vi "Test MIO Digital Measurement.vi"(7 "Config":T1={"Samples to Read (50)"=50, "Channel (0)"=0, "Read Function (Get All)"=enum."Get Latest", "Port(0)"=0}, 8 "error in (no error)":errorcluster, 9 "Instrument":i32, 10 "Test Label":string, 11 "Test Class in":refnum<class "Test Class.lvclass">) -> (0 "error out":errorcluster, 1 "Result":string, 2 "Passed":bool, 3 "Test Class out":refnum<class "Test Class.lvclass">)   [LabVIEW 2015, in "Test Class.lvclass"]
uses:
  Test Class.lvclass
  Digital MIO Measurement Config -- Cluster.ctl
  Classes/Instruments/MIO Device/Class/typedefs/Read Type -- Enum.ctl
  Classes/Instruments/MIO Device/Class/typedefs/Channel Type -- Enum.ctl
  Classes/Instruments/MIO Device/Class/MIO Device.lvclass
  Test Class.lvclass/Test Class.ctl
  Classes/Application/Class/Application.lvclass
  Classes/Test Recipe/Class/Test Recipe.lvclass
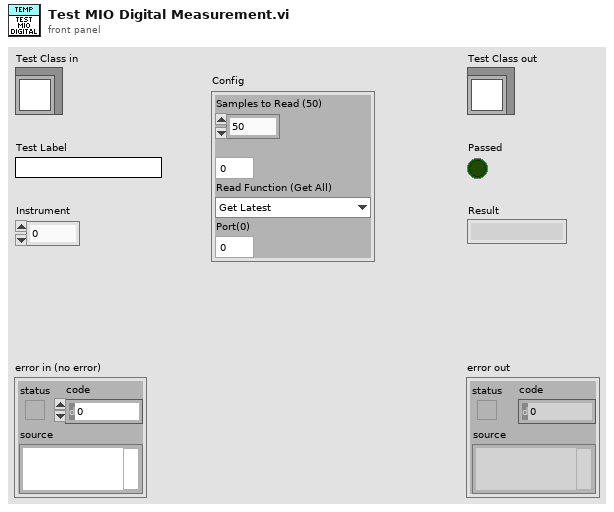
[diagram p1: front panel]
types:
  T1 = typedef "Test Class.lvclass/Digital MIO Measurement Config -- Cluster.ctl" = cluster{"Samples to Read (50)":i32, "Channel (0)":u32, "Read Function (Get All)":T2, "Port(0)":u32}
  T2 = typedef "MIO Device.lvlib/MIO Device.lvclass/Read Type -- Enum.ctl" = enum16{"Get All", "Get Latest", "Get Average"}
  T3 = typedef "MIO Device.lvlib/MIO Device.lvclass/Channel Type -- Enum.ctl" = enum16{"Analog Input", "Analog Output", "Digital Input", "Digital Output"}
  T4 = typedef "Application.lvlib/App Properties.lvclass/Class Properties -- Cluster.ctl" = cluster{"UUT Info":T5[], "Test Information":refnum<vi>, "Test Complete Event":refnum<user-event>, "Shop Floor System":refnum<class "Shop Floor System.lvclass">, "Gold Board":refnum<class "Golden Board.lvclass">, "Test Recipe":refnum<class "Test Recipe.lvclass">, "Instruments":refnum<class "Base Class.lvclass">[], "Mode":T6, "Test Results":cluster{"Pass":bool[], "Fail Codes":string[]}}
  T5 = typedef "Application.lvlib/App Properties.lvclass/UUT Reference -- Cluster.ctl" = cluster{"Serial Number Reference":refnum<vi>, "Status Message Reference":refnum<vi>}
  T6 = typedef "Application.lvlib/Application.lvclass/Op Mode -- Enum.ctl" = u16
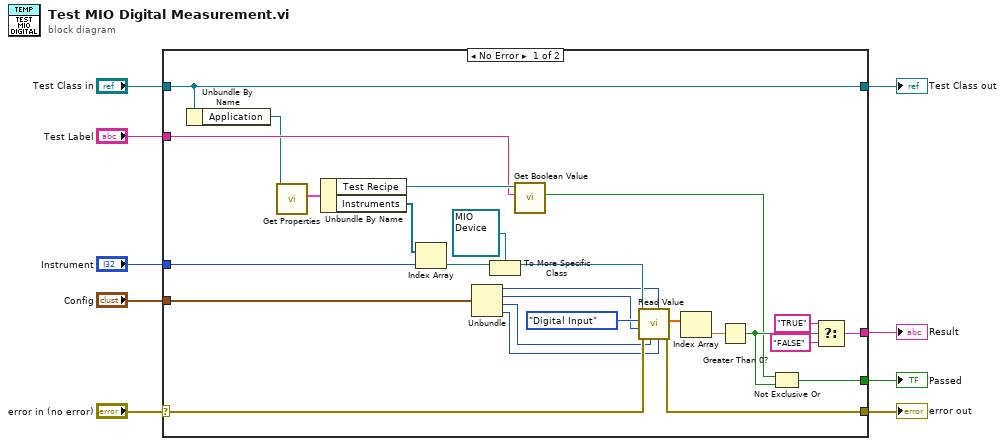
[diagram p0: block diagram]
diagram:
  n1 = case shown="No Error" "error in (no error)" {
    selector: "error in (no error)" -> [w23 w37]
    tunnel: [w22 w37] -> w8
    tunnel: [w26 w36] -> w6
    tunnel: "Test Class in" -> [w26 w36]
    tunnel: "Test Label" -> [w27 _]
    tunnel: [w16 _] -> w4
    tunnel: [w15 _] -> w3
    tunnel: "Instrument" -> [w24 _]
    tunnel: "Config" -> [w14 _]
    frame No Error {
      n2 = Unbundle By Name(w26) -> ("Application"=w25:refnum<class "Application.lvclass">)
      n3 = call "Get Properties.vi"("Acrobat Template in"=w25) -> ("Class Properties"=w33:T4)  [unwired: 8 in, 2 out]
      n4 = Unbundle By Name(w33) -> ("Test Recipe"=w28:refnum<class "Test Recipe.lvclass">, "Instruments"=w34:refnum<class "Base Class.lvclass">[])
      n5 = Index Array(array=w34, index=w24) -> (element=w35:refnum<class "Base Class.lvclass">)
      n6 = Unbundle(w14) -> ("Samples to Read (50)"=w13:i32, "Channel (0)"=w12:u32, "Read Function (Get All)"=w11:T2, "Port(0)"=w10:u32)
      n7 = To More Specific Class(target class=refnum<class "MIO Device.lvclass"> refnum ("MIO Device.lvlib:MIO Device.lvclass"), reference=w35) -> (specific class reference=w32:refnum<class "MIO Device.lvclass">)  [unwired: 1 in, 1 out]
      n8 = call "Get Boolean Value.vi"("Name"=w27, "Test Recipe in"=w28) -> ("Value"=w18:bool)  [unwired: 7 in, 2 out]
      n9 = call-dynamic "Read Value.vi"("Port (0)"=w10, "Samples to Read (50)"=w13, "Read Function (Get All)"=w11, "error in (no error)"=w23, "Channel (0)"=w12, "Channel Type"=Channel_Type_--_Enum."Digital Input", "MIO Device in"=w32) -> ("error out"=w22:errorcluster, "Value"=w30:dbl[])  [unwired: 2 in, 1 out]
      n10 = Index Array(array=w30) -> (element=w17:dbl)  [unwired: 1 in]
      n11 = Greater Than 0?(x=w17) -> (x > 0?=w19:bool)
      n12 = Not Exclusive Or(1:w19, 2:w18) -> (0:w15:bool)
      n13 = Select(t="TRUE", s=w19, f="FALSE") -> (s? t:f=w16:string)
    }
    frame Error {
    }
  }
  "error out" <- w8
  "Test Class out" <- w6
  "Passed" <- w3
  "Result" <- w4
